vi "IIR Cascade Filter with I.C..vi"   [LabVIEW 2024, in "NI_AALBase.lvlib"]
doc: "<p>Filters the input sequence <strong>X</strong> using the cascade form of the IIR filter specified by the <strong>IIR Filter Cluster</strong>. This VI is similar to the <a href=\"nihelplauncher://docs/csh?context=lvcore_lvanls_iir_cascade_filter\">IIR Cascade Filter</a> VI except that you specify the initial conditions for this VI. Wire data to the <strong>X</strong> input to determine the polymorphic instance to use or <a href=\"nihelplauncher://docs/csh?context=lvcore_lvhowto_selectingdefaultinstpolyvi\">manually select</a> the instance.</p>"
uses:
  NI_AALBase.lvlib
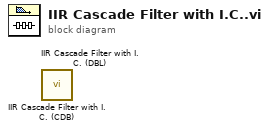
[diagram p0: block diagram]
diagram:
  n1 = call "IIR Cascade Filter with I.C. (CDB).vi"() -> ()  [unwired: 3 in, 3 out]
  n2 = call "IIR Cascade Filter with I.C. (DBL).vi"() -> ()  [unwired: 3 in, 3 out]
